vi "Generate Calibrated Stepped Sine Waveform.vi"(0 "TSM context":T1, 5 "Sweep Configuration":T2[](array[typedef]), 7 "Sample rate":dbl, 9 "Duration in Cycles? (F)":bool, 11 "error in (no error)":errorcluster, 12 "Total Expected Samples":i32=128, 13 "Number Of Sites":i32) -> (4 "PerSite Waveform":waveform(dbl)[](array[waveform]), 6 "Capture Duration":dbl[](array[numeric]), 8 "Frequency":dbl[](array[numeric]), 15 "error out":errorcluster)   [LabVIEW 2020]
doc: "This Vi helps to generate a stepped sine waveform"
uses:
  Typedefs/Acoustic Sweep Config Cluster.ctl
  <vilib>/NI_TestStand_SemiconductorModule/NI_TestStand_Semiconductor_Module.lvlibp/PinMap/General/SemiconductorModuleContext.ctl
  Typedefs/Stepped sine waveform data.ctl
  <vilib>/measure/NI_MABase.lvlib
  <vilib>/NI_TestStand_SemiconductorModule/NI_TestStand_Semiconductor_Module.lvlibp
panel:
  out "Waveform Graph":waveform(dbl)[](graph)
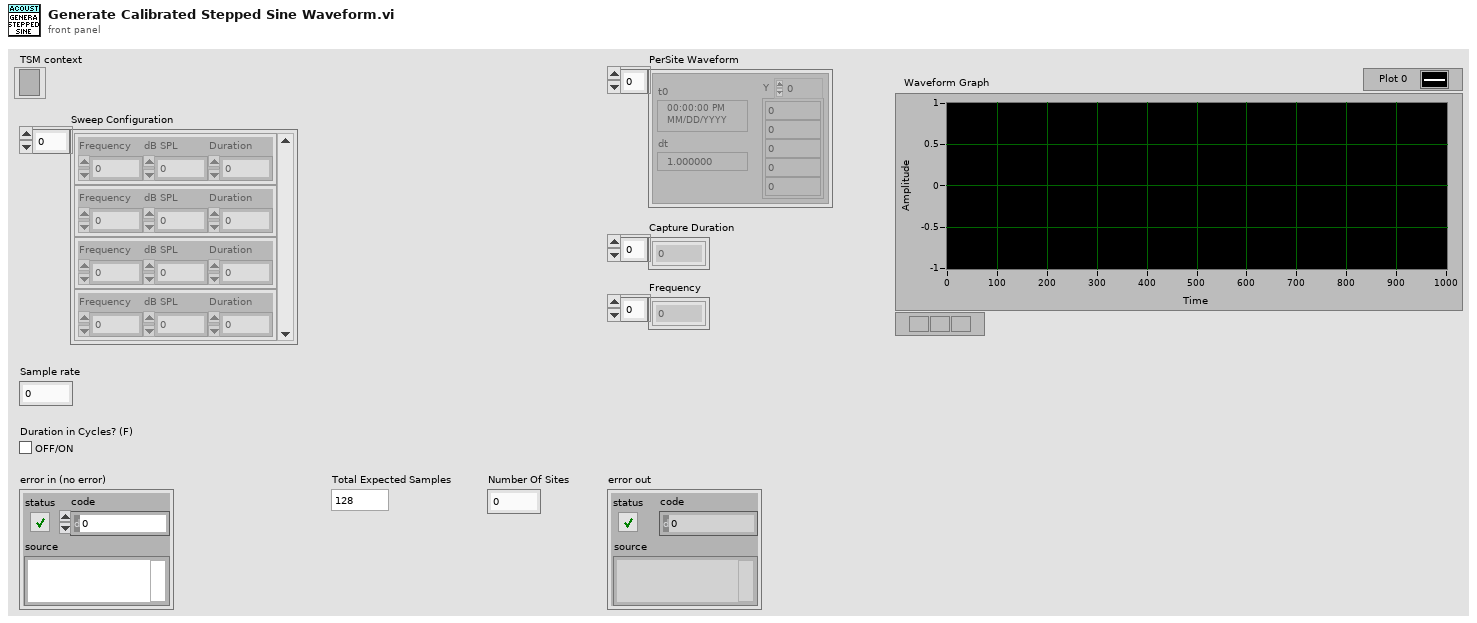
[diagram p1: front panel]
types:
  T1 = typedef "NI_TestStand_Semiconductor_Module.lvlibp/SemiconductorModuleContext.ctl" = refnum<k7>
  T2 = typedef "Acoustic Sweep Config Cluster.ctl" = cluster{"Frequency":dbl, "dB SPL":dbl, "Duration":dbl}
  T3 = typedef "Stepped sine waveform data.ctl" = cluster{"PerSite Waveform":waveform(dbl)[], "Phase":dbl, "SampleCount":i32}
  T4 = enum16{"Sine Wave", "Triangle Wave", "Square Wave", "Sawtooth Wave"}
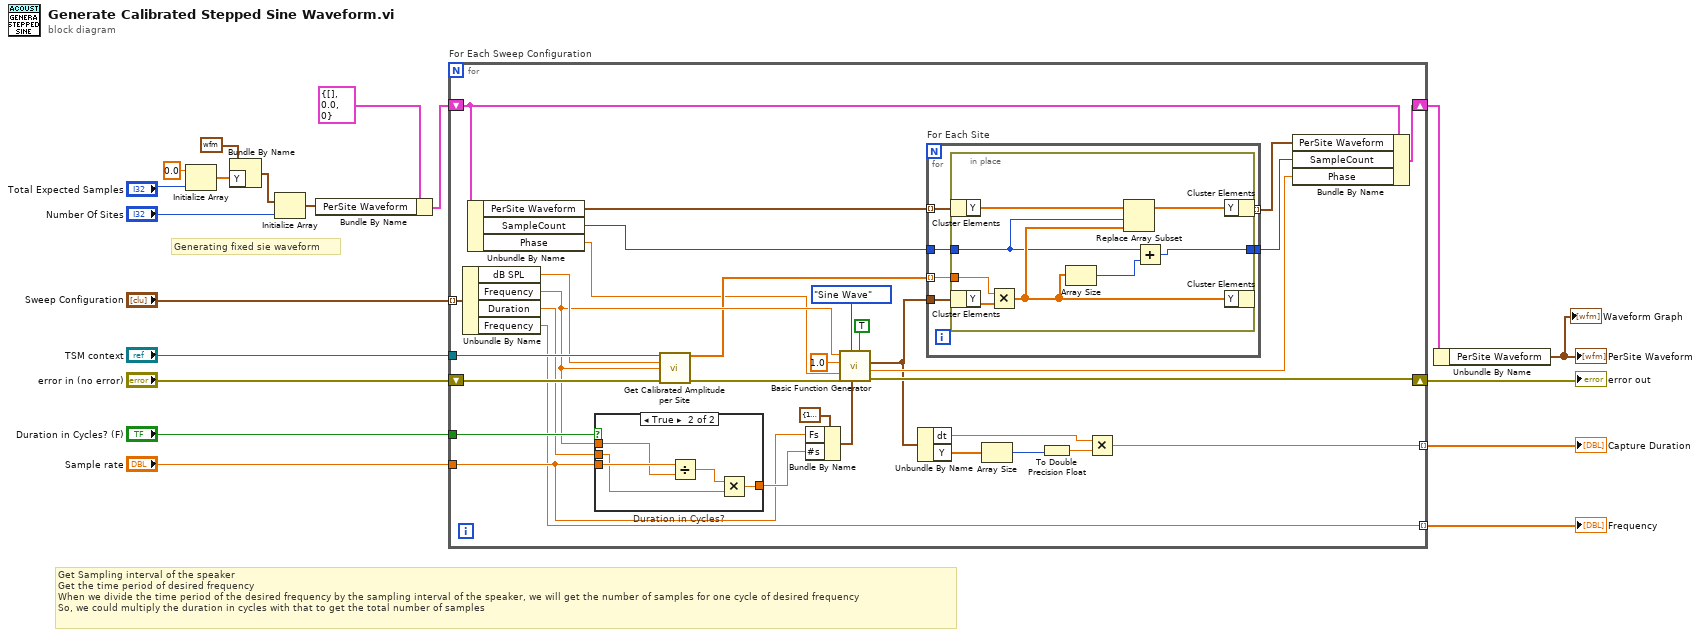
[diagram p0: block diagram]
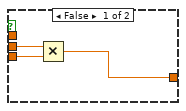
[diagram p2: hidden frame]
diagram:
  # "Get Sampling interval of the speaker \nGet the time period of desired frequency\nWhen we divide the time period of the desired frequency by the sampling interval of the speaker, we will get the number of samples for one cycle of desired frequency\nSo, we could multiply the duration in cycles with that to get the total number of samples"
  # "Generating fixed sie waveform"
  n1 = Initialize Array(0.0, "Total Expected Samples") -> (w8:dbl[])
  n2 = Bundle By Name(cluster=waveform(dbl) {"t0"=timestamp(0 s since 1904-01-01), "dt"=1.0, "Y"=[]} ("Waveform In"), "Y"=w8) -> (w7:waveform(dbl))
  n3 = Initialize Array(w7, "Number Of Sites") -> (w4:waveform(dbl)[])
  n4 = Bundle By Name(cluster=T3 {"PerSite Waveform"=[], "Phase"=0.0, "SampleCount"=0}, "PerSite Waveform"=w4) -> (w2:T3)
  n5 = for "For Each Sweep Configuration" {
    tunnel: "Sweep Configuration" -> [w51] mode=indexing
    tunnel: "TSM context" -> [w49]
    shift-right: [w26] -> w12
    shift-left: "error in (no error)" -> [w48]
    tunnel: "Sample rate" -> [w40]
    tunnel: "Duration in Cycles? (F)" -> [w41]
    shift-right: [w32] -> w14
    shift-left: w2 -> [w33]
    tunnel: [w29] -> w13 mode=indexing
    tunnel: [w20] -> w11 mode=indexing
    n6 = Unbundle By Name(w51) -> ("dB SPL"=w39:dbl, "Frequency"=w38:dbl, "Duration"=w37:dbl, "Frequency"=w29:dbl)
    n7 = Unbundle By Name(w33) -> ("PerSite Waveform"=w34:waveform(dbl)[], "SampleCount"=w28:i32, "Phase"=w35:dbl)
    n8 = case "Duration in Cycles?" shown="True" w41 {
      tunnel: w37 -> [w52 w56]
      tunnel: w40 -> [w54 w59]
      tunnel: [w53 w55] -> w42
      tunnel: w38 -> [_ w58]
      frame False {
        n9 = Multiply(x=w52, y=w54) -> (x*y=w53:dbl)
      }
      frame True {
        n10 = Divide(x=w59, y=w58) -> (x/y=w57:dbl)
        n11 = Multiply(x=w57, y=w56) -> (x*y=w55:dbl)
      }
    }
    n12 = call "Get Calibrated Amplitude per Site.vi"("TSM context"=w49, "dB SPL"=w39, "Frequency (Hz)"=w38, "error in (no error)"=w48) -> ("Per Site Amplitude (V)"=w36:dbl[], "error out"=w46:errorcluster)  [unwired: 9 in, 1 out]
    n13 = Bundle By Name(cluster=cluster{"Fs":dbl, "#s":dbl} {"Fs"=1000.0, "#s"=1000.0} ("sampling info"), "Fs"=w40, "#s"=w42) -> (w43:cluster{"Fs":dbl, "#s":dbl})
    n14 = call <vilib>:"Basic Function Generator.vi"("reset signal"=TRUE, "sampling info"=w43, "signal type"=T4."Sine Wave", "error in (no error)"=w46, "phase"=w35, "amplitude"=1.0, "frequency"=w38) -> ("error out"=w26:errorcluster, "phase out"=w30:dbl, "signal out"=w25:waveform(dbl))  [unwired: 2 in]
    n15 = Unbundle By Name(w25) -> ("dt"=w21:dbl, "Y"=w24:dbl[])
    n16 = for "For Each Site" {
      tunnel: w25 -> [w65]
      tunnel: [w62] -> w31 mode=indexing
      tunnel: w36 -> [w64] mode=indexing
      tunnel: w34 -> [w63] mode=indexing
      tunnel: w28 -> [w61]
      tunnel: [w60] -> w27
      n17 = in-place {
        in-place-border: w64 -> [w72]
        in-place-border: w61 -> [w68]
        in-place-border: [w66] -> w60
        n18 = in-place-cluster #1(w63) -> ("Y"=w71:dbl[])
        n19 = in-place-cluster #2(w65) -> ("Y"=w73:dbl[])
        n20 = Multiply(x=w72, y=w73) -> (x*y=w69:dbl[])
        n21 = Array Size(array=w69) -> (size(s)=w67:i32)
        n22 = Replace Array Subset(array=w71, new element=w69, index=w68) -> (w70:dbl[])
        n23 = Add(x=w68, y=w67) -> (x+y=w66:i32)
        n24 = in-place-cluster #1("Y"=w70) -> (w62:waveform(dbl))
        n25 = in-place-cluster #2("Y"=w69) -> ()  [unwired: 1 out]
      }
    }
    n26 = Array Size(array=w24) -> (size(s)=w23:i32)
    n27 = To Double Precision Float(number=w23) -> (double precision float=w22:dbl)
    n28 = Multiply(x=w21, y=w22) -> (x*y=w20:dbl)
    n29 = Bundle By Name(cluster=w33, "PerSite Waveform"=w31, "SampleCount"=w27, "Phase"=w30) -> (w32:T3)
  }
  "error out" <- w12
  "Capture Duration" <- w11
  "Frequency" <- w13
  n30 = Unbundle By Name(w14) -> ("PerSite Waveform"=→"PerSite Waveform" →"Waveform Graph":waveform(dbl)[])
